vi "GetCamera.vi"(3 "error out 2":errorcluster) -> (12 "CCD Chip horizontal end":i32, 14 "CCD Chip Vertical end":i32, 16 "array":i32[][](array[numeric]), 17 "error out":errorcluster, 18 "low":i32, 19 "high":i32, 27 "kinetic":sgl format="%.2f")   [LabVIEW 2013]
uses:
  Variables/GlobalSetGetConfigureCamera.vi
  Variables/ccdChipPixels.vi
  lib/atmcd32d.llb/ReadMode_mode typedef.ctl
  lib/atmcd32d.llb/AcquisitionMode_mode typedef.ctl
  lib/atmcd32d.llb/TriggerMode_mode typedef.ctl
  lib/atmcd32d.llb/Shutter_type typedef.ctl
  lib/atmcd32d.llb/Shutter_mode typedef.ctl
  lib/atmcd32d.llb/HSSpeed_type typedef.ctl
  lib/atmcd32d.llb/EMGainMode_mode typedef.ctl
  C:/Users/user/Desktop/AbelFCS/Camera/lib/atmcd32d.llb/Error Code Enum typedef.ctl
  lib/atmcd32d.llb/Spool_method typedef.ctl
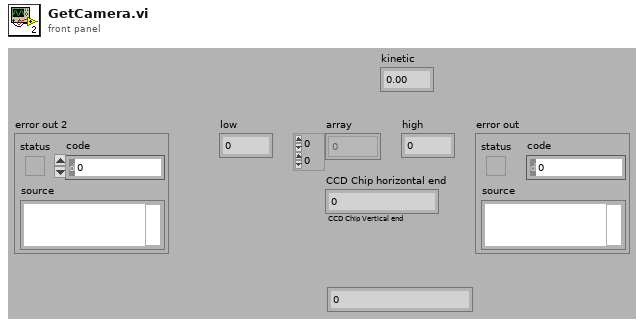
[diagram p1: front panel]
types:
  T1 = typedef "Spool_method typedef.ctl" = enum16{"32-bit", "Depends", "16-bit", "Multiple Directory", "Spool to RAM disk", "16-bit FITS", "SIF", "16-buit TIFF", "Multiple Directory Compressed"}
  T2 = typedef "EMGainMode_mode typedef.ctl" = enum16{"8-bit", "12-bit", "Linear", "Real"}
  T3 = typedef "HSSpeed_type typedef.ctl" = enum16{"EM Amp", "Conventional Amp"}
  T4 = typedef "Shutter_mode typedef.ctl" = enum16{"Auto", "Open", "Close"}
  T5 = typedef "Shutter_type typedef.ctl" = enum16{"TTL Low", "TTL High"}
  T6 = typedef "TriggerMode_mode typedef.ctl" = enum16{"Internal", "External", "N/A (2)", "N/A (3)", "N/A (4)", "N/A (5)", "External Start"}
  T7 = typedef "AcquisitionMode_mode typedef.ctl" = enum16{"Reserved (0)", "Single Scan", "Accumulate", "Kinetics", "Fast Kinetics", "Run Till Abort", "Reserved (6)", "Reserved (7)", "Reserved (8)", "Time Delayed Integration"}
  T8 = typedef "ReadMode_mode typedef.ctl" = enum16{"Full Vertical Binning", "Multi-Track", "Random-Track", "Single-Track", "Image"}
  T9 = typedef "Error Code Enum typedef.ctl" = enum32{"N/A (0)", "DRV_ERROR_CODES", "DRV_SUCCESS", "DRV_VXDNOTINSTALLED", "DRV_ERROR_SCAN", "DRV_ERROR_CHECK_SUM", "DRV_ERROR_FILELOAD", "DRV_UNKNOWN_FUNC", "DRV_ERROR_VXD_INIT", "DRV_ERROR_ADDRESS", "DRV_ERROR_PAGELOCK", "DRV_ERROR_PAGEUNLOCK", "DRV_ERROR_BOARDTEST", "DRV_ERROR_ACK", "DRV_ERROR_UP_FIFO", "DRV_ERROR_PATTERN", "N/A (16)", "DRV_ACQUISITION_ERRORS", "DRV_ACQ_BUFFER", "DRV_ACQ_DOWNFIFO_FULL", "DRV_PROC_UNKONWN_INSTRUCTION", "DRV_ILLEGAL_OP_CODE", "DRV_KINETIC_TIME_NOT_MET", "DRV_ACCUM_TIME_NOT_MET", "DRV_NO_NEW_DATA", "N/A (25)", "DRV_SPOOLERROR", "N/A (27)", "N/A (28)", "N/A (29)", "N/A (30)", "N/A (31)", "N/A (32)", "DRV_TEMPERATURE_CODES", "DRV_TEMPERATURE_OFF", "DRV_TEMPERATURE_NOT_STABILIZED", "DRV_TEMPERATURE_STABILIZED", "DRV_TEMPERATURE_NOT_REACHED", "DRV_TEMPERATURE_OUT_RANGE", "DRV_TEMPERATURE_NOT_SUPPORTED", "DRV_TEMPERATURE_DRIFT", "N/A (41)", "N/A (42)", "N/A (43)", "N/A (44)", "N/A (45)", "N/A (46)", "N/A (47)", "N/A (48)", "DRV_GENERAL_ERRORS", "DRV_INVALID_AUX", "DRV_COF_NOTLOADED", "DRV_FPGAPROG", "DRV_FLEXERROR", "DRV_GPIBERROR", "N/A (55)", "N/A (56)", "N/A (57)", "N/A (58)", "N/A (59)", "N/A (60)", "N/A (61)", "N/A (62)", "N/A (63)", "DRV_DATATYPE", "DRV_DRIVER_ERRORS", "DRV_P1INVALID", "DRV_P2INVALID", "DRV_P3INVALID", "DRV_P4INVALID", "DRV_INIERROR", "DRV_COFERROR", "DRV_ACQUIRING", "DRV_IDLE", "DRV_TEMPCYCLE", "DRV_NOT_INITIALIZED", "DRV_P5INVALID", "DRV_P6INVALID", "DRV_INVALID_MODE", "DRV_INVALID_FILTER", "DRV_I2CERRORS", "DRV_I2CDEVNOTFOUND", "DRV_I2CTIMEOUT", "DRV_P7INVALID", "N/A (84)", "N/A (85)", "N/A (86)", "N/A (87)", "N/A (88)", "N/A (89)", "DRV_IOCERROR", "DRV_VRMVERSIONERROR"}
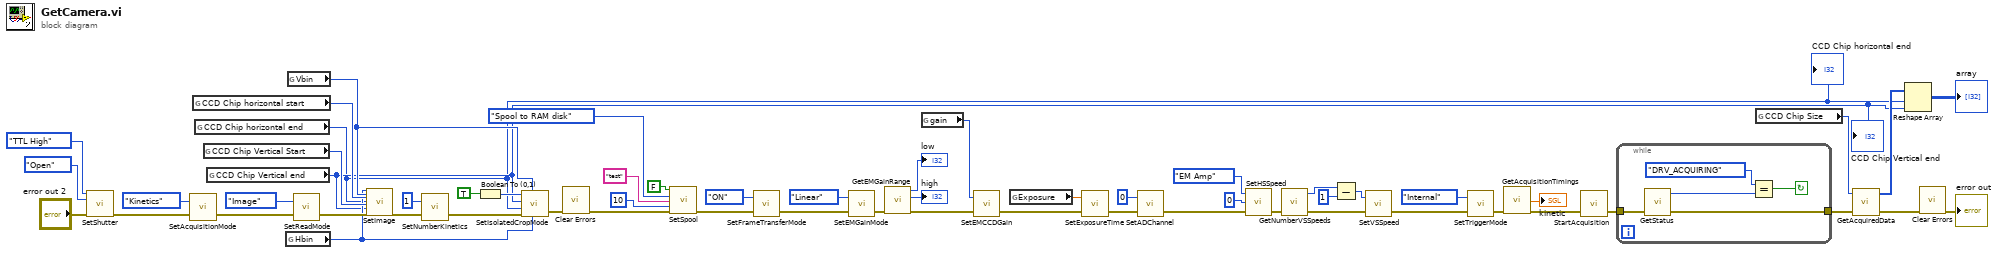
[diagram p0: block diagram]
diagram:
  n1 = call "SetShutter.vi"("type"=Shutter_type_typedef."TTL High", "mode"=Shutter_mode_typedef."Open", "error in (no error)"="error out 2") -> ("error out"=w53:errorcluster)  [unwired: 11 in, 1 out]
  n2 = call "SetAcquisitionMode.vi"("error in (no error)"=w53, "mode"=AcquisitionMode_mode_typedef."Kinetics") -> ("error out"=w29:errorcluster)  [unwired: 1 out]
  n3 = global read "ccdChipPixels.vi" "CCD Chip horizontal start"() -> (w27:i32)
  n4 = global read "ccdChipPixels.vi" "CCD Chip horizontal end"() -> (w10:i32)
  "CCD Chip horizontal end" <- w10
  n5 = global read "ccdChipPixels.vi" "CCD Chip Vertical Start"() -> (w28:i32)
  n6 = global read "ccdChipPixels.vi" "CCD Chip Vertical end"() -> (w11:i32)
  "CCD Chip Vertical end" <- w11
  n7 = global read "GlobalSetGetConfigureCamera.vi" "Hbin"() -> (w12:i32)
  n8 = global read "GlobalSetGetConfigureCamera.vi" "Vbin"() -> (w13:i32)
  n9 = call "SetReadMode.vi"("error in (no error)"=w29, "mode"=ReadMode_mode_typedef."Image") -> ("error out"=w30:errorcluster)  [unwired: 1 out]
  n10 = call "SetImage.vi"("hbin"=w12, "vbin"=w13, "hstart"=w27, "hend"=w10, "vstart"=w28, "vend"=w11, "error in (no error)"=w30) -> ("error out"=w57:errorcluster)  [unwired: 19 in, 1 out]
  n11 = call "SetNumberKinetics.vi"("error in (no error)"=w57, "number"=1) -> ("error out"=w16:errorcluster)  [unwired: 1 out]
  n12 = Boolean To (0,1)(Boolean=TRUE) -> (0, 1=w17:i16)
  n13 = call "SetIsolatedCropMode.vi"("hbin"=w12, "vbin"=w13, "error in (no error)"=w16, "cropWidth"=w10, "cropHeight"=w11, "active"=w17) -> ("error out"=w9:errorcluster)  [unwired: 1 out]
  n14 = call <vilib>:"Clear Errors.vi"("error in (no error)"=w9) -> ("error out"=w8:errorcluster)  [unwired: 6 in]
  n15 = call "SetSpool.vi"("active"=FALSE, "method"=Spool_method_typedef."Spool to RAM disk", "name"="test", "framebuffersize (10)"=10, "error in (no error)"=w8) -> ("error out"=w15:errorcluster)  [unwired: 9 in, 1 out]
  n16 = call "SetFrameTransferMode.vi"("error in (no error)"=w15, "mode"=enum16{"OFF", "ON"}."ON") -> ("error out"=w14:errorcluster)  [unwired: 1 out]
  n17 = call "SetEMGainMode.vi"("error in (no error)"=w14, "mode"=EMGainMode_mode_typedef."Linear") -> ("error out"=w49:errorcluster)  [unwired: 1 out]
  n18 = call "GetEMGainRange.vi"("error in (no error)"=w49) -> ("error out"=w50:errorcluster, "high"=→"high":i32, "low"=→"low":i32)  [unwired: 3 in, 1 out]
  n19 = global read "GlobalSetGetConfigureCamera.vi" "gain"() -> (w26:i32)
  n20 = call "SetEMCCDGain.vi"("error in (no error)"=w50, "gain"=w26) -> ("error out"=w48:errorcluster)  [unwired: 1 out]
  n21 = global read "GlobalSetGetConfigureCamera.vi" "Exposure"() -> (w25:sgl)
  n22 = call "SetExposureTime.vi"("error in (no error)"=w48, "time"=w25) -> ("error out"=w31:errorcluster)  [unwired: 1 out]
  n23 = call "SetADChannel.vi"("error in (no error)"=w31, "channel"=0) -> ("error out"=w32:errorcluster)  [unwired: 1 out]
  n24 = call "SetHSSpeed.vi"("error in (no error)"=w32, "index"=0, "type"=HSSpeed_type_typedef."EM Amp") -> ("error out"=w36:errorcluster)  [unwired: 1 in, 1 out]
  n25 = call "GetNumberVSSpeeds.vi"("error in (no error)"=w36) -> ("error out"=w38:errorcluster, "number"=w35:i32)  [unwired: 2 in, 1 out]
  n26 = Subtract(x=w35, y=1) -> (x-y=w33:i32)
  n27 = call "SetVSSpeed.vi"("error in (no error)"=w38, "index"=w33) -> ("error out"=w37:errorcluster)  [unwired: 1 out]
  n28 = call "SetTriggerMode.vi"("error in (no error)"=w37, "mode"=TriggerMode_mode_typedef."Internal") -> ("error out"=w4:errorcluster)  [unwired: 1 out]
  n29 = call "GetAcquisitionTimings.vi"("error in (no error)"=w4) -> ("kinetic"=→"kinetic":sgl, "error out"=w3:errorcluster)  [unwired: 10 in, 3 out]
  n30 = call "StartAcquisition.vi"("error in (no error)"=w3) -> ("error out"=w7:errorcluster)  [unwired: 1 in, 1 out]
  n31 = while {
    tunnel: w7 -> [w63]
    tunnel: [w62] -> w6
    stop <- w59 continue-if-true
    n32 = call "GetStatus.vi"("error in (no error)"=w63) -> ("error out"=w62:errorcluster, "status"=w60:T9)  [unwired: 2 in, 1 out]
    n33 = Equal?(x=Error_Code_Enum_typedef."DRV_ACQUIRING" ("status"), y=w60) -> (x = y?=w59:bool)
  }
  n34 = global read "ccdChipPixels.vi" "CCD Chip Size"() -> (w1:i32)
  n35 = call "GetAcquiredData.vi"("error in (no error)"=w6, "size"=w1) -> ("error out"=w5:errorcluster, "array"=w24:i32[])  [unwired: 1 in, 1 out]
  n36 = Reshape Array(w24, w10, w11) -> (→"array":i32[][])
  n37 = call <vilib>:"Clear Errors.vi"("error in (no error)"=w5) -> ("error out"=→"error out":errorcluster)  [unwired: 6 in]
